vi "Set_Output_State.vi"(3 "rest off?":bool, 4 "error in":errorcluster, 5 "channel":u8=2 min=2 max=13 step=1, 6 "state":bool=TRUE, 7 "VISA arduino in":refnum<visa-resource-name>) -> (0 "error out":errorcluster, 1 "VISA arduino out":refnum<visa-resource-name>)   [LabVIEW 2021]
uses:
  Delay_Global.vi
  <vilib>/Utility/error.llb/Error Cluster From Error Code.vi
  <vilib>/ErrorRing/Error Ring.xnode
panel:
  out "delay":u32
  # "Private"
  # "Public"
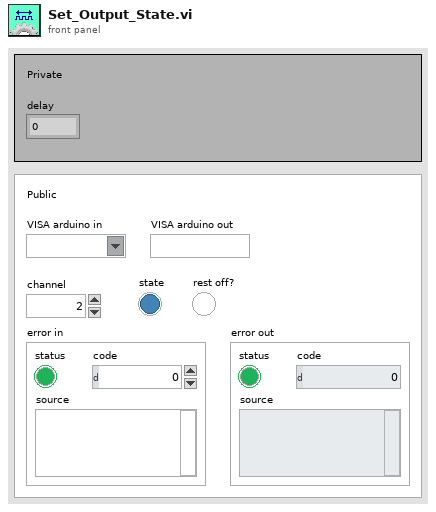
[diagram p1: front panel]
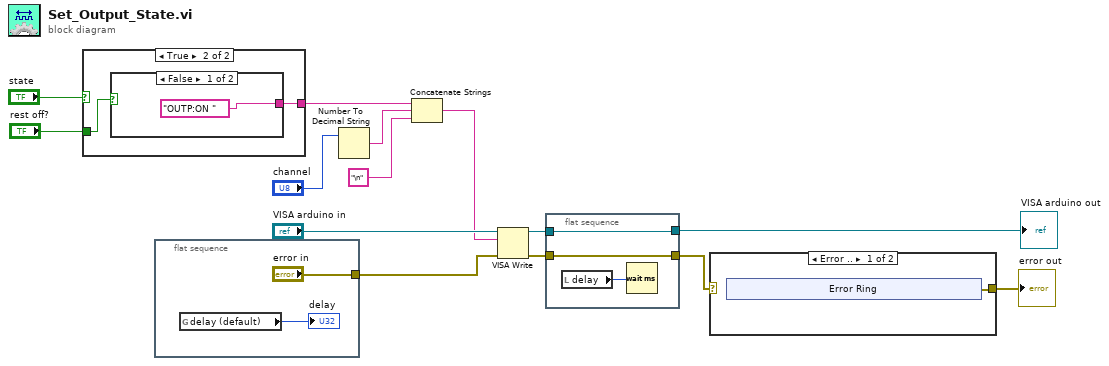
[diagram p0: block diagram]
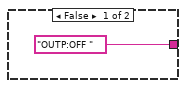
[diagram p3: hidden frame]
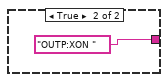
[diagram p4: hidden frame]
diagram:
  n1 = case shown="True" "state" {
    tunnel: "rest off?" -> [_ w17]
    tunnel: ["OUTP:OFF " w16] -> w11
    frame False {
    }
    frame True {
      n2 = case shown="False" w17 {
        tunnel: ["OUTP:ON " "OUTP:XON "] -> w16
        frame False {
        }
        frame True {
        }
      }
    }
  }
  n3 = flat-sequence {
    tunnel: ["error in"] -> w7
    frame #0 {
      n4 = global read "Delay_Global.vi" "delay (default)"() -> (→"delay":u32)
    }
  }
  n5 = Number To Decimal String(number="channel") -> (decimal integer string=w10:string)  [unwired: 1 in]
  n6 = Concatenate Strings(w11, w10, "\n" ("string")) -> (w6:string)
  n7 = VISA Write(VISA resource name="VISA arduino in", write buffer=w6, error in (no error)=w7) -> (VISA resource name out=w5:refnum<visa-resource-name>, error out=w4:errorcluster)  [unwired: 1 out]
  n8 = flat-sequence {
    tunnel: w5 -> [w23]
    tunnel: w4 -> [w22]
    tunnel: [w23] -> w2
    tunnel: [w22] -> w3
    frame #0 {
      n9 = local read "delay"() -> (w24:u32)
      n10 = Wait (ms)(milliseconds to wait=w24) -> ()  [unwired: 1 out]
    }
  }
  n11 = case shown="Error .." w3 {
    selector: w3 -> [_ w31]
    tunnel: [w25 w31] -> w1
    frame Error {
      n12 = xnode "Error Ring"() -> ("error out"=w25:errorcluster)
    }
    frame No Error {
    }
  }
  "error out" <- w1
  "VISA arduino out" <- w2
